vi "Motor_UpdateInput(Angle).vi"(5 "Enabled":bool[](array[boolean]), 7 "CableTensionNow(N)":dbl[](array[numeric]), 8 "error in (no error)":errorcluster, 9 "MotorShaftSpeed(rad/s)":dbl[](array[numeric]), 10 "MotorEncAngle(rad)":dbl[](array[numeric]), 11 "Motor in":refnum<class "MotorControl.lvclass">) -> (0 "error out":errorcluster, 3 "Motor out":refnum<class "MotorControl.lvclass">)   [LabVIEW 2015, in "MotorControl.lvclass"]
uses:
  MotorControl.lvclass
  MotorControl.lvclass/MotorControl.ctl
  <vilib>/ptbypt/NI_PtbyPt.lvlib
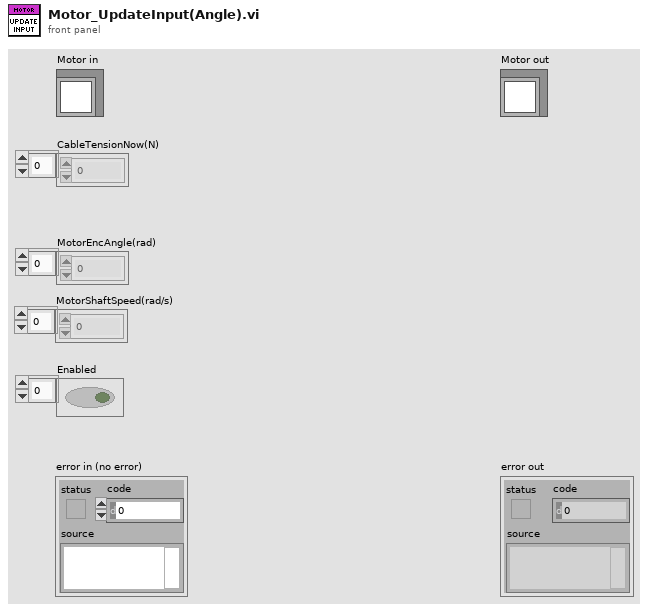
[diagram p1: front panel]
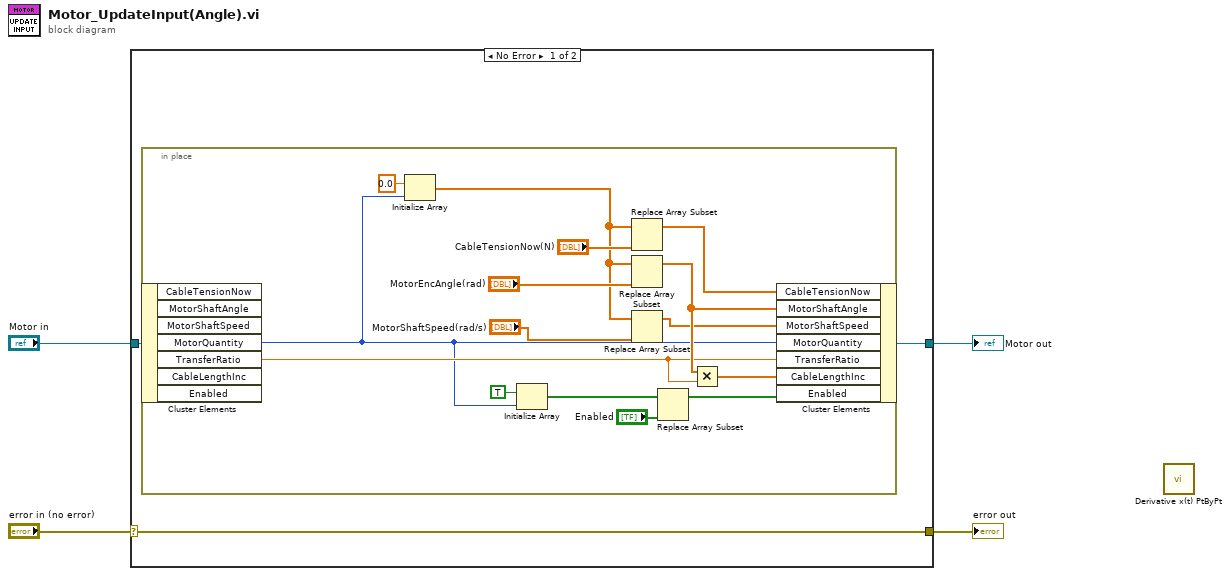
[diagram p0: block diagram]
diagram:
  n1 = case shown="No Error" "error in (no error)" {
    selector: "error in (no error)" -> [w5 w24]
    tunnel: [w5 w24] -> w3
    tunnel: [w6 w23] -> w1
    tunnel: "Motor in" -> [w7 w23]
    frame No Error {
      n2 = in-place {
        n3 = in-place-cluster #1(w7) -> ("MotorQuantity"=w16:i32, "TransferRatio"=w18:dbl)  [unwired: 5 out]
        n4 = Initialize Array(0.0 ("element"), w16) -> (w9:dbl[])
        n5 = Initialize Array(TRUE, w16) -> (w14:bool[])
        n6 = Replace Array Subset(array=w9, new element="CableTensionNow(N)") -> (w17:dbl[])  [unwired: 1 in]
        n7 = Replace Array Subset(array=w9, new element="MotorEncAngle(rad)") -> (w20:dbl[])  [unwired: 1 in]
        n8 = Replace Array Subset(array=w9, new element="MotorShaftSpeed(rad/s)") -> (w10:dbl[])  [unwired: 1 in]
        n9 = Replace Array Subset(array=w14, new element="Enabled") -> (w11:bool[])  [unwired: 1 in]
        n10 = Multiply(x=w20, y=w18) -> (x*y=w19:dbl[])
        n11 = in-place-cluster #1("CableTensionNow"=w17, "MotorShaftAngle"=w20, "MotorShaftSpeed"=w10, "MotorQuantity"=w16, "TransferRatio"=w18, "CableLengthInc"=w19, "Enabled"=w11) -> (w6:refnum<class "MotorControl.lvclass">)
      }
    }
    frame Error {
    }
  }
  "error out" <- w3
  "Motor out" <- w1
  n12 = call <vilib>:"Derivative x(t) PtByPt.vi"() -> ()  [unwired: 4 in, 2 out]
